vi "Write Parity Bit.vi"(8 "error in":errorcluster, 11 "32-bit word in":refnum<class "32-bit Word.lvclass">) -> (0 "error out":errorcluster, 3 "32-bit word out":refnum<class "32-bit Word.lvclass">)   [LabVIEW 2020, in "32-bit Word.lvclass"]
uses:
  32-bit Word.lvclass
  C:/Git/niveristand-communications-bus-template/Source/Protocol/Implementations/ARINC429/ARINC 429.lvclass
  ARINC 429.lvclass/ARINC 429.ctl
  32-bit Word.lvclass/32-bit Word.ctl
  bb557d58-e434-4093-9d62-477f60b714fb.vi
  Read Parity.vi
  Read 32-Bit Word.vi
  Read Parity Index.vi
  Write 32-Bit Word.vi
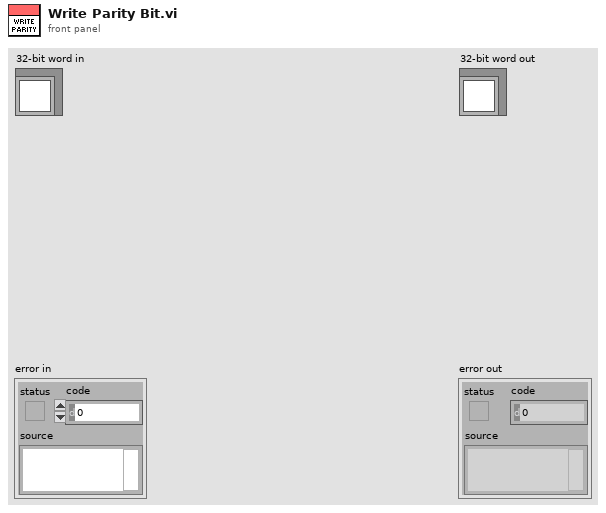
[diagram p1: front panel]
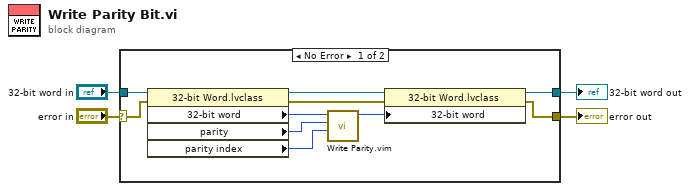
[diagram p0: block diagram]
diagram:
  n1 = case shown="No Error" "error in" {
    selector: "error in" -> [w12 w16]
    tunnel: [w9 w16] -> w3
    tunnel: [w13 w15] -> w1
    tunnel: "32-bit word in" -> [w11 w15]
    frame No Error {
      n2 = property class="32-bit Word.lvclass"(reference=w11, error in=w12) -> (reference out=w14:refnum<class "32-bit Word.lvclass">, error out=w10:errorcluster, "32-bit word"=w7:u32, "parity"=w6:enum16{"Even", "Odd"}, "parity index"=w5:i32)
      n3 = call "Write Parity.vim"("parity index"=w5, "parity"=w6, "32-bit word in"=w7) -> ("32-bit word out"=w8:u32)  [unwired: 8 in]
      n4 = property class="32-bit Word.lvclass"(reference=w14, error in=w10, "32-bit word"=w8) -> (reference out=w13:refnum<class "32-bit Word.lvclass">, error out=w9:errorcluster)
    }
    frame Error {
    }
  }
  "error out" <- w3
  "32-bit word out" <- w1
